vi "rangchange.vi"(3 "datafile":path[](array[path]), 4 "savaen":bool, 5 "IN":i32[](array[numeric]), 6 "添加的数组 2":T1(array[ring])) -> (1 "添加的数组":dbl[][](array[numeric]))   [LabVIEW 2012]
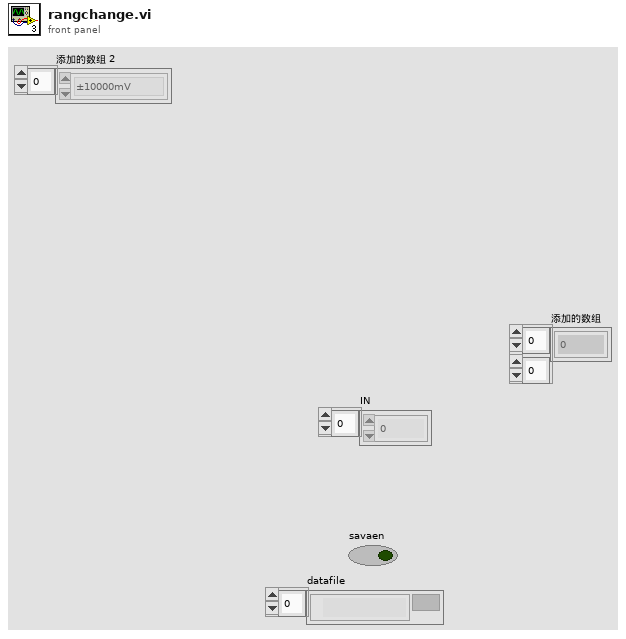
[diagram p1: front panel]
types:
  T1 = enum16{"±10000mV", "±5000mV", "±2500mV", "0-10000mV", "0-5000mV"}[]
  T2 = enum16{"±10000mV", "±5000mV", "±2500mV", "0-10000mV", "0-5000mV"}
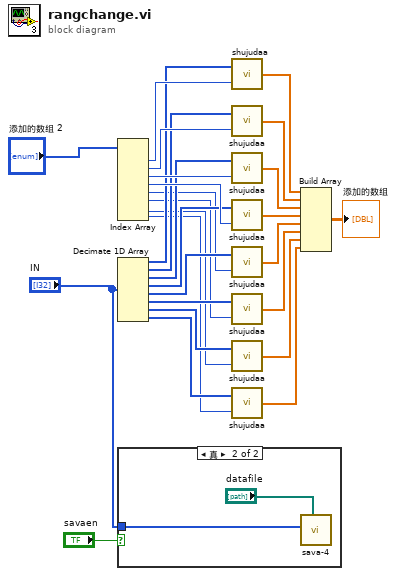
[diagram p0: block diagram]
diagram:
  n1 = Index Array(array="添加的数组 2") -> (element #1=w28:T2, element #2=w27:T2, element #3=w26:T2, element #4=w25:T2, element #5=w15:T2, element #6=w14:T2, element #7=w13:T2, element #8=w12:T2)  [unwired: 8 in]
  n2 = Decimate 1D Array("IN") -> (w24:i32[], w23:i32[], w22:i32[], w21:i32[], w19:i32[], w18:i32[], w17:i32[], w16:i32[])
  n3 = case shown="真" "savaen" {
    tunnel: "IN" -> [_ w29]
    frame False {
    }
    frame True {
      n4 = call "sava-4.vi"("datafile"="datafile", "1D array"=w29) -> ()  [unwired: 10 in]
    }
  }
  n5 = call "shujudaa.vi"("量程-1"=w28, "inputdata"=w24) -> ("outdata"=w11:dbl[])
  n6 = call "shujudaa.vi"("量程-1"=w27, "inputdata"=w23) -> ("outdata"=w10:dbl[])
  n7 = call "shujudaa.vi"("量程-1"=w26, "inputdata"=w22) -> ("outdata"=w9:dbl[])
  n8 = call "shujudaa.vi"("量程-1"=w25, "inputdata"=w21) -> ("outdata"=w8:dbl[])
  n9 = call "shujudaa.vi"("量程-1"=w15, "inputdata"=w19) -> ("outdata"=w7:dbl[])
  n10 = call "shujudaa.vi"("量程-1"=w14, "inputdata"=w18) -> ("outdata"=w6:dbl[])
  n11 = call "shujudaa.vi"("量程-1"=w13, "inputdata"=w17) -> ("outdata"=w5:dbl[])
  n12 = call "shujudaa.vi"("量程-1"=w12, "inputdata"=w16) -> ("outdata"=w4:dbl[])
  n13 = Build Array(w11, w10, w9, w8, w7, w6, w5, w4) -> (→"添加的数组":dbl[][])
